vi "Raycaster_ReadWallHeight.vi"(9 "Sub Buffer Address":u32, 10 "Sub Buffer":u8, 11 "Frame Buffers In":T1) -> (2 "Height":i16, 3 "Frame Buffers Out":T1)   [LabVIEW 2020]
uses:
  Controls/Raycaster_DrawState.ctl
  <vilib>/rvi/DataTransferAndStorage/Container/XNode/niFpgaContainer.xnode
  <vilib>/rvi/Memory/Memory_Emulation/nirvimemoryEmulation.vi
  <vilib>/rvi/Memory/Memory_Emulation/nirvimemoryFastEmulation.vi
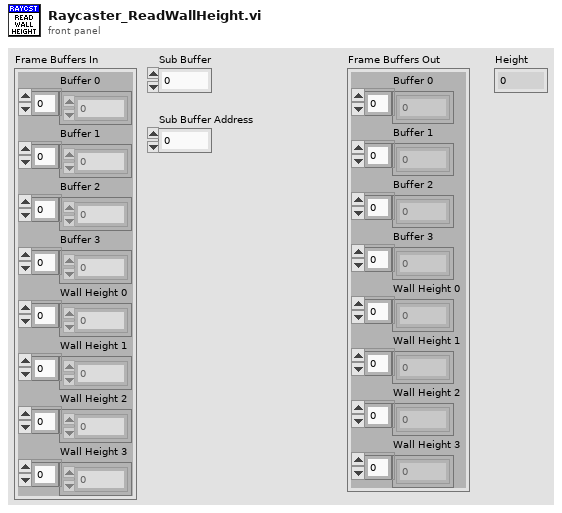
[diagram p1: front panel]
types:
  T1 = typedef "Raycaster_DrawState.ctl" = cluster{"Buffer 0":u8[], "Buffer 1":u8[], "Buffer 2":u8[], "Buffer 3":u8[], "Wall Height 0":i16[], "Wall Height 1":i16[], "Wall Height 2":i16[], "Wall Height 3":i16[]}
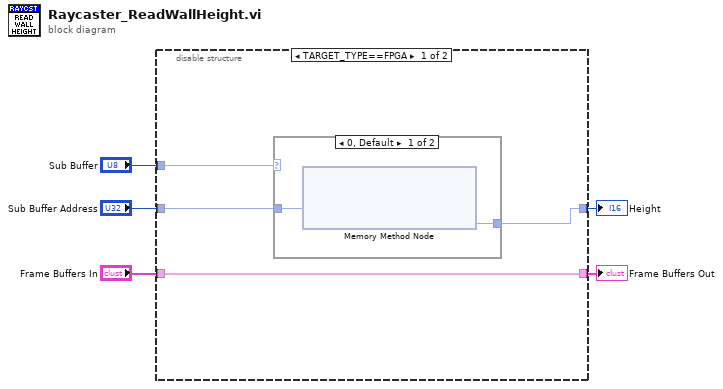
[diagram p0: block diagram]
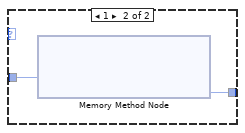
[diagram p2: hidden frame]
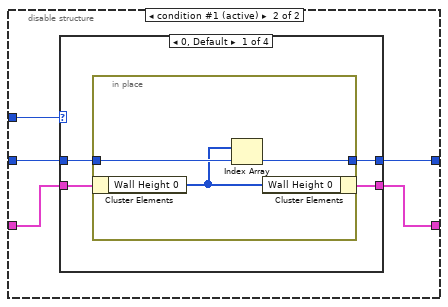
[diagram p3: hidden frame]
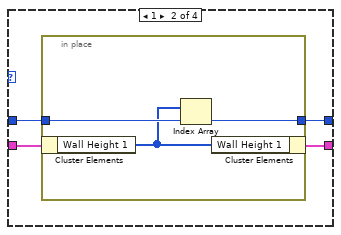
[diagram p4: hidden frame]
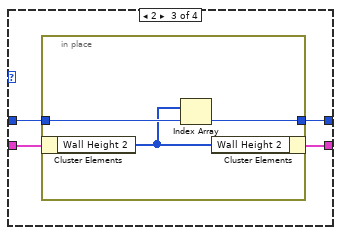
[diagram p5: hidden frame]
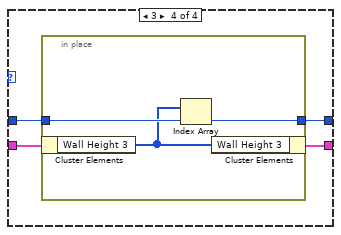
[diagram p6: hidden frame]
diagram:
  n1 = disable-structure shown="TARGET_TYPE==FPGA" {
    disable-tunnel: "Sub Buffer" -> [w7 w18]
    disable-tunnel: "Sub Buffer Address" -> [w9 w17]
    disable-tunnel: "Frame Buffers In" -> [w8 w16]
    disable-tunnel: [w8 w15] -> w2
    disable-tunnel: [w6 w14] -> w1
    frame condition #0 {
      n2 = case shown="0, Default" w7 {
        tunnel: w9 -> [w11 w13]
        tunnel: [w10 w12] -> w6
        frame 0, Default {
          n3 = xnode ("Memory Method Node")("Address"=w11) -> ("Data"=w10:i16)  [unwired: 1 in, 1 out]
        }
        frame 1 {
          n4 = xnode ("Memory Method Node")("Address"=w13) -> ("Data"=w12:i16)  [unwired: 1 in, 1 out]
        }
      }
    }
    frame condition #1 (active) {
      n5 = case shown="0, Default" w18 {
        tunnel: w16 -> [w22 w29 w36 w43]
        tunnel: w17 -> [w21 w28 w35 w42]
        tunnel: [w20 w27 w34 w41] -> w15
        tunnel: [w19 w26 w33 w40] -> w14
        frame 0, Default {
          n6 = in-place {
            in-place-border: w21 -> [w25]
            in-place-border: [w23] -> w19
            n7 = in-place-cluster #1(w22) -> ("Wall Height 0"=w24:i16[])
            n8 = Index Array(array=w24, index=w25) -> (element=w23:i16)
            n9 = in-place-cluster #1("Wall Height 0"=w24) -> (w20:T1)
          }
        }
        frame 1 {
          n10 = in-place {
            in-place-border: w28 -> [w32]
            in-place-border: [w30] -> w26
            n11 = in-place-cluster #2(w29) -> ("Wall Height 1"=w31:i16[])
            n12 = Index Array(array=w31, index=w32) -> (element=w30:i16)
            n13 = in-place-cluster #2("Wall Height 1"=w31) -> (w27:T1)
          }
        }
        frame 2 {
          n14 = in-place {
            in-place-border: w35 -> [w39]
            in-place-border: [w37] -> w33
            n15 = in-place-cluster #3(w36) -> ("Wall Height 2"=w38:i16[])
            n16 = Index Array(array=w38, index=w39) -> (element=w37:i16)
            n17 = in-place-cluster #3("Wall Height 2"=w38) -> (w34:T1)
          }
        }
        frame 3 {
          n18 = in-place {
            in-place-border: w42 -> [w46]
            in-place-border: [w44] -> w40
            n19 = in-place-cluster #4(w43) -> ("Wall Height 3"=w45:i16[])
            n20 = Index Array(array=w45, index=w46) -> (element=w44:i16)
            n21 = in-place-cluster #4("Wall Height 3"=w45) -> (w41:T1)
          }
        }
      }
    }
  }
  "Frame Buffers Out" <- w2
  "Height" <- w1
